vi "Read Currents.vi"(0 "Session Handle":T1, 11 "error in (no error)":errorcluster) -> (4 "Session Handle Out":T1, 6 "Side 1 Current":dbl, 8 "Side 2 Current":dbl, 15 "error out":errorcluster)   [LabVIEW 2015, in "Peltier.lvclass"]
uses:
  Peltier.lvclass
  Typedefs/Session Handle.ctl
  Gas/Gas.lvclass
panel:
  out "Success?":bool
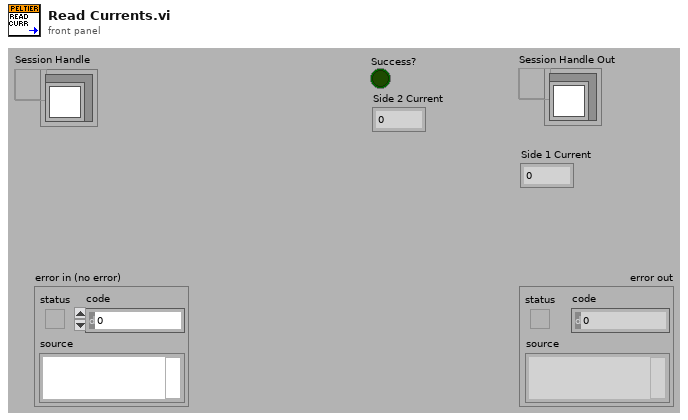
[diagram p1: front panel]
types:
  T1 = typedef "Peltier.lvclass/Session Handle.ctl" = refnum<data-value>
  T2 = typedef "XNET Frame CAN.ctl" = cluster{"timestamp":timestamp, "payload":u8[], "identifier":u32, "type":T3, "extended?":bool, "echo?":bool}
  T3 = typedef "XNET Frame Type CAN.ctl" = u8
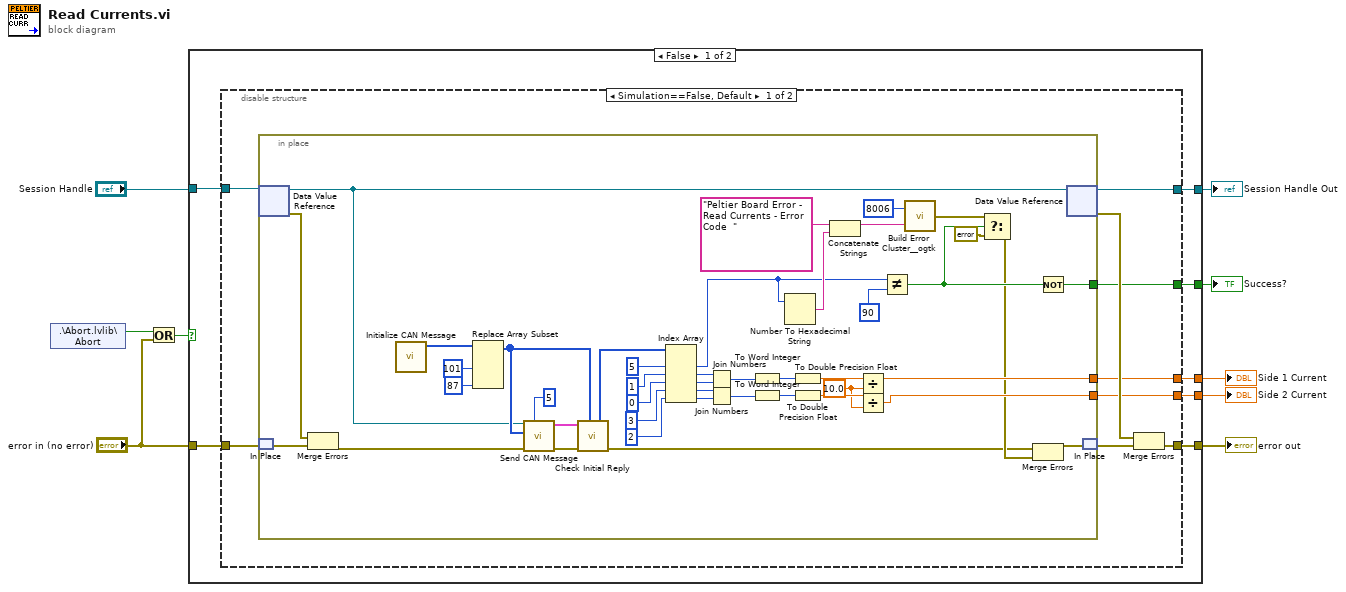
[diagram p0: block diagram]
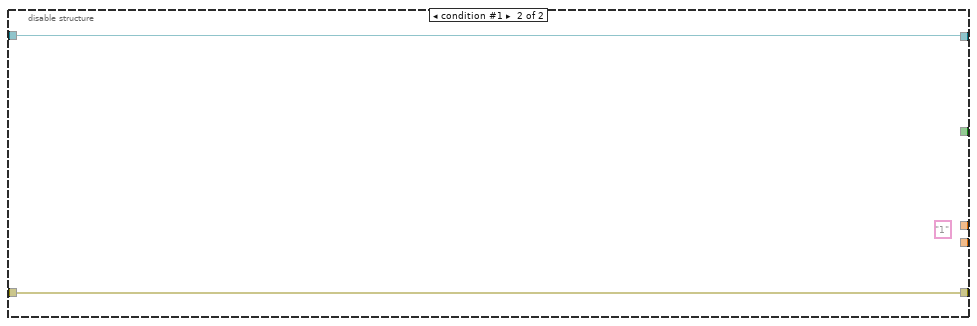
[diagram p2: hidden frame]
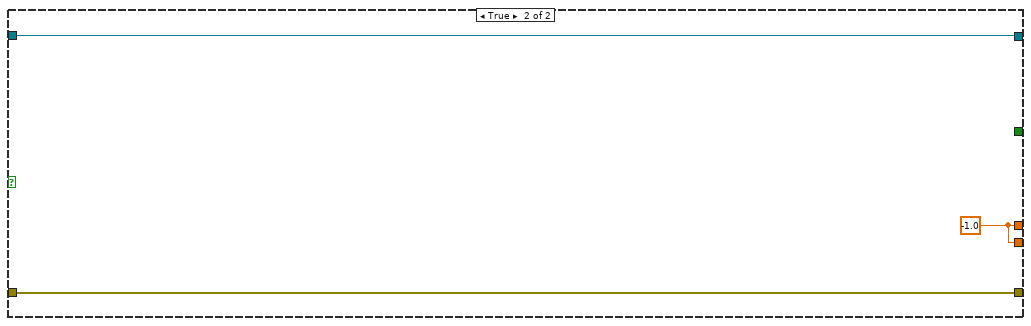
[diagram p3: hidden frame]
diagram:
  n1 = shared-variable ".\\Abort.lvlib\\Abort"() -> (w8:bool)  [unwired: 1 in, 1 out]
  n2 = Or(x=w8, y="error in (no error)") -> (x .or. y?=w6:bool)
  n3 = case shown="False" w6 {
    tunnel: [w16 w73] -> w2
    tunnel: [w15 w72] -> w9
    tunnel: "Session Handle" -> [w14 w73]
    tunnel: "error in (no error)" -> [w13 w72]
    tunnel: [w12 w71] -> w5
    tunnel: [w11 _] -> w4
    tunnel: [w10 w71] -> w1
    frame False {
      n4 = disable-structure shown="Simulation==False, Default" {
        disable-tunnel: [w25 w70] -> w16
        disable-tunnel: [w22 w69] -> w15
        disable-tunnel: w14 -> [w21 w70]
        disable-tunnel: w13 -> [w20 w69]
        disable-tunnel: [w19 _] -> w12
        disable-tunnel: [w18 _] -> w11
        disable-tunnel: [w17 _] -> w10
        frame condition #0 (active) {
          n5 = in-place {
            in-place-border: [w32] -> w19
            in-place-border: [w50] -> w18
            in-place-border: [w29] -> w17
            w30 = 10.0 ("y")
            n6 = in-place-dvr #1(w21) -> (w59:refnum<class "Peltier.lvclass">, w64:errorcluster)
            n7 = in-place-match #2(w20) -> (w63:errorcluster)
            n8 = Merge Errors(w64, w63) -> (w58:errorcluster)
            n9 = call "Initialize CAN Message.vi"() -> ("Initial Payload"=w66:u8[])  [unwired: 11 in]
            n10 = Replace Array Subset(array=w66, new element #1=u8 101 ("new element/subarray"), new element #2=u8 87 ("new element/subarray")) -> (w62:u8[])  [unwired: 2 in]
            n11 = call "Send CAN Message.vi"("Number of Retries"=5, "error in (no error)"=w58, "payload"=w62, "Peltier In"=w59) -> ("error out"=w27:errorcluster, "Reply"=w60:T2[])  [unwired: 5 in, 1 out]
            n12 = call "Check Initial Reply.vi"("Write Message"=w62, "error in (no error)"=w27, "Reply"=w60) -> ("error out"=w26:errorcluster, "Data Packet"=w65:u8[])  [unwired: 5 in, 2 out]
            n13 = Index Array(array=w65, index #1=5 ("index"), index #2=1 ("index"), index #3=0 ("index"), index #4=3 ("index"), index #5=2 ("index")) -> (element #1=w51:u8, element #2=w46:u8, element #3=w45:u8, element #4=w36:u8, element #5=w35:u8)
            n14 = Join Numbers(hi=w46, lo=w45) -> ((hi.lo)=w44:u16)
            n15 = Join Numbers(hi=w36, lo=w35) -> ((hi.lo)=w38:u16)
            n16 = To Word Integer(number=w44) -> (16bit integer=w47:i16)
            n17 = To Word Integer(number=w38) -> (16bit integer=w37:i16)
            n18 = Number To Hexadecimal String(2:w51) -> (0:w55:string)  [unwired: 1 in]
            n19 = To Double Precision Float(number=w47) -> (double precision float=w34:dbl)
            n20 = To Double Precision Float(number=w37) -> (double precision float=w31:dbl)
            n21 = Concatenate Strings("Peltier Board Error -  Read Currents - Error Code  " ("string"), w55) -> (w54:string)
            n22 = Divide(x=w34, y=w30) -> (x/y=w32:dbl)
            n23 = Divide(x=w31, y=w30) -> (x/y=w29:dbl)
            n24 = Not Equal?(x=w51, y=u8 90 ("new element/subarray")) -> (x != y?=w41:bool)
            n25 = call <userlib>:"Build Error Cluster__ogtk.vi"("String to Prepend to source (\"\")"=w54, "code"=8006) -> ("error out"=w43:errorcluster)
            n26 = Select(t=w43, s=w41, f=errorcluster {"status"=FALSE, "code"=0, "source"=""}) -> (s? t:f=w28:errorcluster)
            n27 = Merge Errors(w26, w28) -> (w67:errorcluster)
            n28 = Not(x=w41) -> (.not. x?=w50:bool)
            n29 = in-place-dvr #1(w59) -> (w25:T1, w23:errorcluster)
            n30 = in-place-match #2(w67) -> (w24:errorcluster)
          }
          n31 = Merge Errors(w23, w24) -> (w22:errorcluster)
        }
        frame condition #1 {
          (unwired) "1"
        }
      }
    }
    frame True {
      w71 = -1.0
    }
  }
  "error out" <- w9
  "Side 1 Current" <- w5
  "Success?" <- w4
  "Session Handle Out" <- w2
  "Side 2 Current" <- w1
